vi "Sequencer - Create Sequence.vi"(0 "Error In":errorcluster) -> (8 "Error Out":errorcluster)   [LabVIEW 2011]
uses:
  <vilib>/Utility/file.llb/Read From Spreadsheet File (string).vi
  <vilib>/Utility/file.llb/Write To Spreadsheet File (string).vi
  Controls/Init-Write-Read.ctl
panel:
  in  "Tab":enum32{"EDIT", "RUN"}(tab)
  in  "BG Process":bool
  in  "Ready":bool
  in  "Load":bool
  in  "Save Button":bool
  in  "Stop Button":bool
  in  "Remove Step":bool
  in  "Down Button":bool
  in  "Up Button":bool
  in  "Add Step":bool
  in  "Sequence":i32(listbox)=1
  in  "Steps":i32(listbox)=1
  in  "NewStep":bool
  in  "Confirm Sequence":i32(listbox)=1
  in  "Cancel":bool
  in  "Run":bool
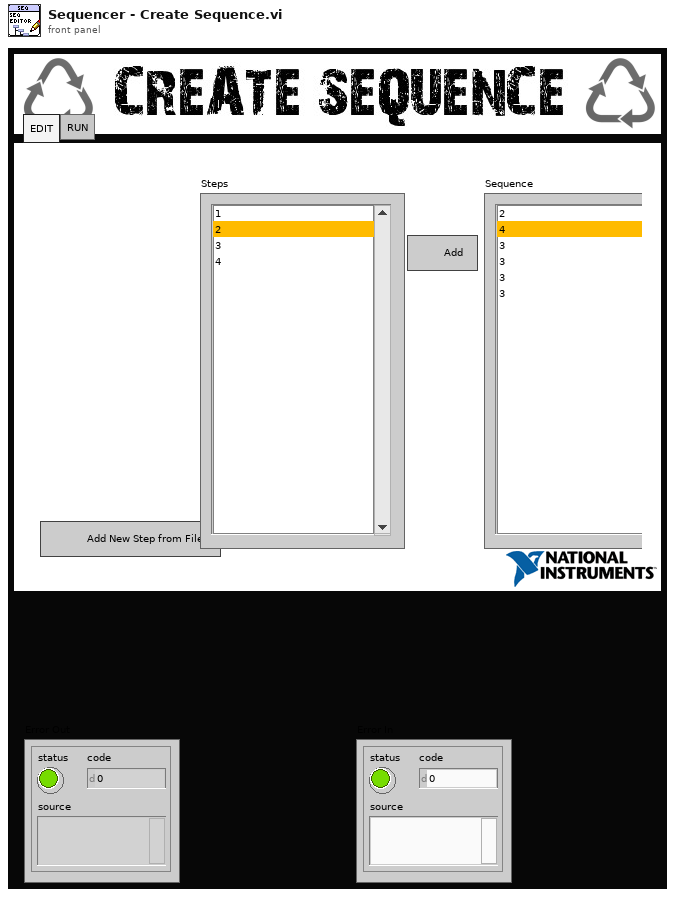
[diagram p1: front panel]
types:
  T1 = typedef "Init-Write-Read.ctl" = enum16{"INIT", "WRITE", "READ", "READ ALL"}
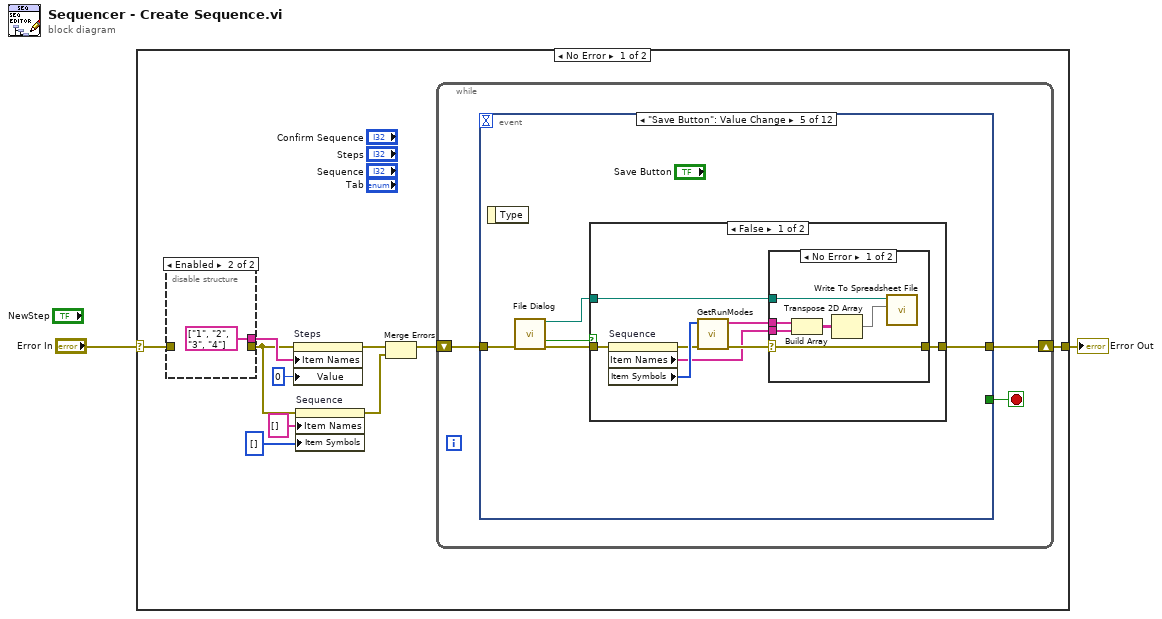
[diagram p0: block diagram]
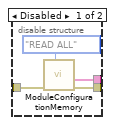
[diagram p2: hidden frame]
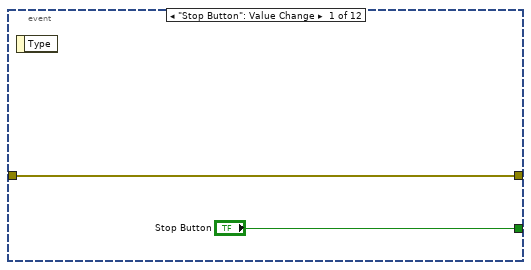
[diagram p3: hidden frame]
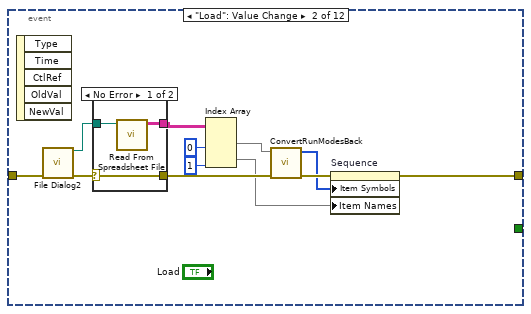
[diagram p4: hidden frame]
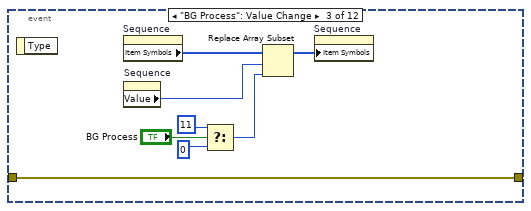
[diagram p6: hidden frame]
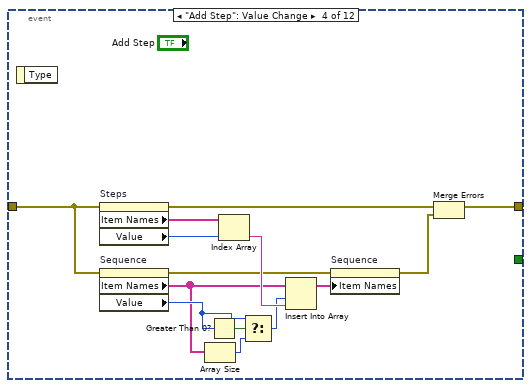
[diagram p7: hidden frame]
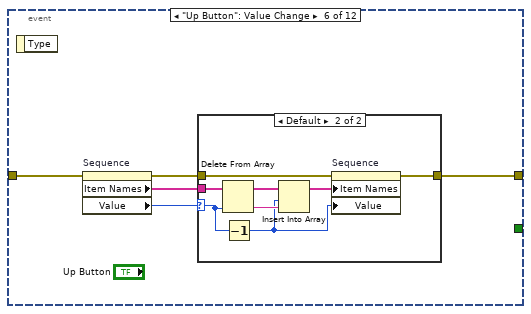
[diagram p10: hidden frame]
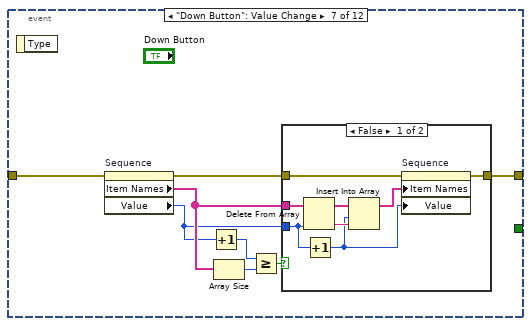
[diagram p12: hidden frame]
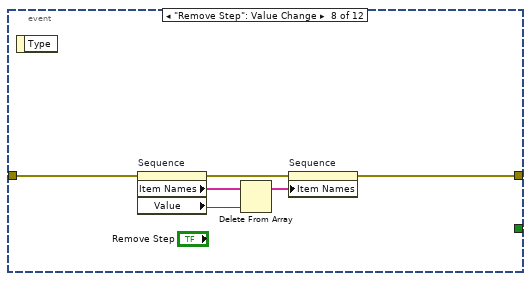
[diagram p14: hidden frame]
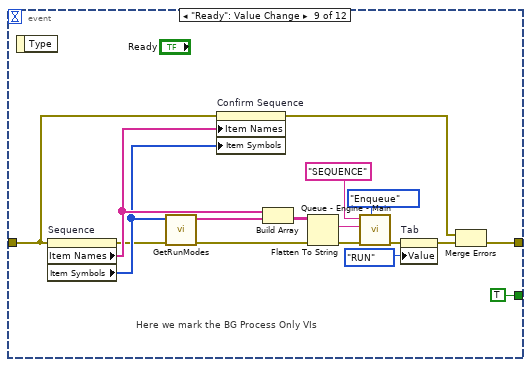
[diagram p15: hidden frame]
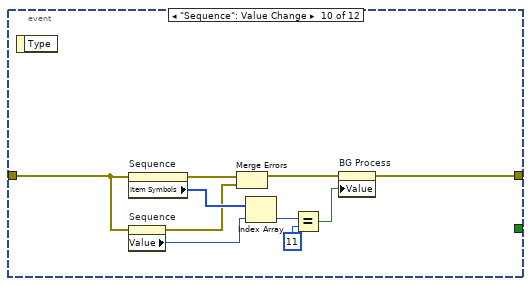
[diagram p16: hidden frame]
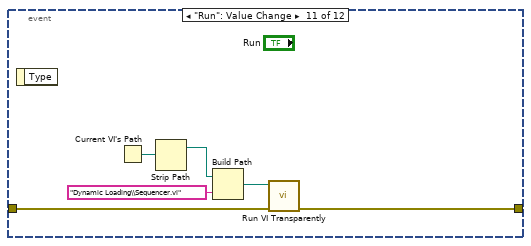
[diagram p17: hidden frame]
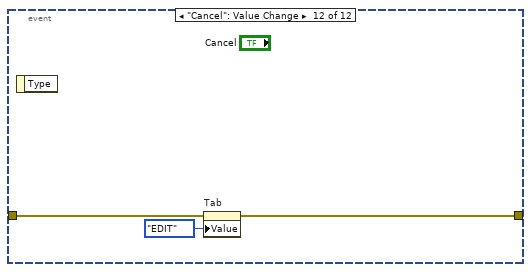
[diagram p18: hidden frame]
diagram:
  n1 = case shown="No Error" "Error In" {
    selector: "Error In" -> [w4 w155]
    tunnel: [w5 w155] -> w2
    frame No Error {
      n2 = disable-structure shown="Enabled" {
        disable-tunnel: [w16 string[] ["1", "2", "3", "4"] ("All Variables Out")] -> w10
        disable-tunnel: [w15 _] -> w9
        disable-tunnel: w4 -> [w14 _]
        frame Disabled {
          n3 = call "ModuleConfigurationMemory.vi"("Operation"=Init-Write-Read."READ ALL", "Error In"=w14) -> ("Error Out"=w15:errorcluster, "All Variables Out"=w16:string[])  [unwired: 5 in, 3 out]
        }
        frame Enabled {
        }
      }
      n4 = property on="Steps" class="LstBox (strict)"(error in=w9, "Item Names"=w10, "Value"=0 ("Steps")) -> (error out=w8:errorcluster)  [unwired: 1 in, 1 out]
      n5 = property on="Sequence" class="LstBox (strict)"(error in=w9, "Item Names"=string[] [], "Item Symbols"=i32[] []) -> (error out=w6:errorcluster)  [unwired: 1 in, 1 out]
      n6 = Merge Errors(w8, w6) -> (w7:errorcluster)
      n7 = while {
        shift-right: [w18] -> w5
        shift-left: w7 -> [w19]
        stop <- w20 stop-if-true
        n8 = event shown="[4] \"Save Button\": Value Change" {
          selector: _ -> [_ _ _ _ _ _ _ _ _ _ _ _]
          dyn-events: _ -> [_ _ _ _ _ _ _ _ _ _ _ _]
          timeout: _ -> [_ _ _ _ _ _ _ _ _ _ _ _]
          tunnel: ["Stop Button" _ _ _ _ _ _ _ TRUE ("Stop Button") _ _ _] -> w20
          tunnel: w19 -> [w21 w31 w43 w51 w62 w83 w97 w114 w126 w140 w151 w153]
          tunnel: [w21 w34 w43 w47 w61 w82 w96 w113 w124 w139 w150 w152] -> w18
          event "Stop Button": Value Change {
            n9 = event-data() -> ()  [unwired: 1 in, 1 out]
          }
          event "Load": Value Change {
            n10 = event-data() -> ()  [unwired: 1 in, 5 out]
            n11 = call "File Dialog2"("error in"=w31) -> ("selected path"=w28:path, "error out"=w30:errorcluster)  [unwired: 11 in, 2 out]
            n12 = case shown="No Error" w30 {
              selector: w30 -> [w37 w38]
              tunnel: [w37 w38] -> w29
              tunnel: w28 -> [w36 _]
              tunnel: [w35 _] -> w27
              frame No Error {
                n13 = call-poly <vilib>:"Read From Spreadsheet File.vi"("file path (dialog if empty)"=w36) -> ("all rows"=w35:string[][])  [unwired: 6 in, 4 out]
              }
              frame Error {
              }
            }
            n14 = Index Array(array=w27, index (col) #1=0 ("disabled index (col)"), index (col) #2=1 ("disabled index (col)")) -> (element #1=w24:string[], element #2=w23:string[])  [unwired: 2 in]
            n15 = call "ConvertRunModesBack.vi"("Error In"=w29, "Run Modes in"=w24) -> ("Error Out"=w33:errorcluster, "Item Symbols Out"=w32:i32[])  [unwired: 8 in]
            n16 = property on="Sequence" class="LstBox (strict)"(error in=w33, "Item Symbols"=w32, "Item Names"=w23) -> (error out=w34:errorcluster)  [unwired: 1 in, 1 out]
          }
          event "BG Process": Value Change {
            n17 = event-data() -> ()  [unwired: 1 in, 1 out]
            n18 = property on="Sequence" class="LstBox (strict)"() -> ("Item Symbols"=w46:i32[])  [unwired: 2 in, 2 out]
            n19 = property on="Sequence" class="LstBox (strict)"() -> ("Value"=w45:i32)  [unwired: 2 in, 2 out]
            n20 = Select(t=11 ("y"), s="BG Process", f=0) -> (s? t:f=w39:i32)
            n21 = Replace Array Subset(array=w46, new element=w39, index=w45) -> (w44:i32[])
            n22 = property on="Sequence" class="LstBox (strict)"("Item Symbols"=w44) -> ()  [unwired: 2 in, 2 out]
          }
          event "Add Step": Value Change {
            n23 = event-data() -> ()  [unwired: 1 in, 1 out]
            n24 = property on="Steps" class="LstBox (strict)"(error in=w51) -> (error out=w49:errorcluster, "Item Names"=w60:string[], "Value"=w59:i32)  [unwired: 1 in, 1 out]
            n25 = property on="Sequence" class="LstBox (strict)"(error in=w51) -> (error out=w50:errorcluster, "Item Names"=w53:string[], "Value"=w55:i32)  [unwired: 1 in, 1 out]
            n26 = Array Size(array=w53) -> (size(s)=w52:i32)
            n27 = Greater Than 0?(x=w55) -> (x > 0?=w56:bool)
            n28 = Index Array(array=w60, index=w59) -> (element=w58:string)
            n29 = Select(t=w55, s=w56, f=w52) -> (s? t:f=w54:i32)
            n30 = Insert Into Array(array=w53, index=w54, new element=w58) -> (w57:string[])
            n31 = property on="Sequence" class="LstBox (strict)"(error in=w50, "Item Names"=w57) -> (error out=w48:errorcluster)  [unwired: 1 in, 1 out]
            n32 = Merge Errors(w49, w48) -> (w47:errorcluster)
          }
          event "Save Button": Value Change {
            n33 = event-data() -> ()  [unwired: 1 in, 1 out]
            n34 = call "File Dialog"("error in"=w62) -> ("selected path"=w63:path, "cancelled"=w65:bool, "error out"=w64:errorcluster)  [unwired: 11 in, 1 out]
            n35 = case shown="False" w65 {
              tunnel: w64 -> [w73 w81]
              tunnel: w63 -> [w68 _]
              tunnel: [w69 w81] -> w61
              frame False {
                n36 = property on="Sequence" class="LstBox (strict)"(error in=w73) -> (error out=w71:errorcluster, "Item Names"=w66:string[], "Item Symbols"=w72:i32[])  [unwired: 1 in, 1 out]
                n37 = call "GetRunModes.vi"("Error In"=w71, "Item Symbols In"=w72) -> ("Error Out"=w70:errorcluster, "Run Modes Out"=w67:string[])  [unwired: 8 in]
                n38 = case shown="No Error" w70 {
                  selector: w70 -> [w79 w80]
                  tunnel: [w79 w80] -> w69
                  tunnel: w68 -> [w78 _]
                  tunnel: w67 -> [w77 _]
                  tunnel: w66 -> [w76 _]
                  frame No Error {
                    n39 = Build Array(w77, w76) -> (w75:string[][])
                    n40 = Transpose 2D Array(2D array=w75) -> (transposed array=w74:string[][])
                    n41 = call-poly <vilib>:"Write To Spreadsheet File.vi"("2D data"=w74, "file path (dialog if empty)"=w78) -> ()  [unwired: 6 in, 1 out]
                  }
                  frame Error {
                  }
                }
              }
              frame True {
              }
            }
          }
          event "Up Button": Value Change {
            n42 = event-data() -> ()  [unwired: 1 in, 1 out]
            n43 = property on="Sequence" class="LstBox (strict)"(error in=w83) -> (error out=w85:errorcluster, "Item Names"=w86:string[], "Value"=w84:i32)  [unwired: 1 in, 1 out]
            n44 = case shown="Default" w84 {
              selector: w84 -> [_ w89]
              tunnel: w86 -> [_ w95]
              tunnel: w85 -> [w87 w91]
              tunnel: [w87 w88] -> w82
              frame 0 {
              }
              frame Default {
                n45 = Delete From Array(array=w95, index=w89) -> (deleted portion=w93:string, array with subset deleted=w94:string[])  [unwired: 1 in]
                n46 = Decrement(x=w89) -> (x-1=w90:i32)
                n47 = Insert Into Array(array=w94, index=w90, new element=w93) -> (w92:string[])
                n48 = property on="Sequence" class="LstBox (strict)"(error in=w91, "Item Names"=w92, "Value"=w90) -> (error out=w88:errorcluster)  [unwired: 1 in, 1 out]
              }
            }
          }
          event "Down Button": Value Change {
            n49 = event-data() -> ()  [unwired: 1 in, 1 out]
            n50 = property on="Sequence" class="LstBox (strict)"(error in=w97) -> (error out=w103:errorcluster, "Item Names"=w102:string[], "Value"=w100:i32)  [unwired: 1 in, 1 out]
            n51 = Increment(x=w100) -> (x+1=w98:i32)
            n52 = Array Size(array=w102) -> (size(s)=w101:i32)
            n53 = Greater Or Equal?(x=w98, y=w101) -> (x >= y?=w99:bool)
            n54 = case shown="False" w99 {
              tunnel: w103 -> [w109 w112]
              tunnel: w102 -> [w108 _]
              tunnel: w100 -> [w106 _]
              tunnel: [w104 w112] -> w96
              frame False {
                n55 = Delete From Array(array=w108, index=w106) -> (deleted portion=w110:string, array with subset deleted=w111:string[])  [unwired: 1 in]
                n56 = Increment(x=w106) -> (x+1=w107:i32)
                n57 = Insert Into Array(array=w111, index=w107, new element=w110) -> (w105:string[])
                n58 = property on="Sequence" class="LstBox (strict)"(error in=w109, "Item Names"=w105, "Value"=w107) -> (error out=w104:errorcluster)  [unwired: 1 in, 1 out]
              }
              frame True {
              }
            }
          }
          event "Remove Step": Value Change {
            n59 = event-data() -> ()  [unwired: 1 in, 1 out]
            n60 = property on="Sequence" class="LstBox (strict)"(error in=w114) -> (error out=w116:errorcluster, "Item Names"=w118:string[], "Value"=w115:i32)  [unwired: 1 in, 1 out]
            n61 = Delete From Array(array=w118, index=w115) -> (array with subset deleted=w117:string[])  [unwired: 1 in, 1 out]
            n62 = property on="Sequence" class="LstBox (strict)"(error in=w116, "Item Names"=w117) -> (error out=w113:errorcluster)  [unwired: 1 in, 1 out]
          }
          event "Ready": Value Change {
            # "Here we mark the BG Process Only VIs"
            n63 = event-data() -> ()  [unwired: 1 in, 1 out]
            n64 = property on="Sequence" class="LstBox (strict)"(error in=w126) -> (error out=w120:errorcluster, "Item Names"=w127:string[], "Item Symbols"=w122:i32[])  [unwired: 1 in, 1 out]
            n65 = call "GetRunModes.vi"("Error In"=w120, "Item Symbols In"=w122) -> ("Error Out"=w119:errorcluster, "Run Modes Out"=w121:string[])  [unwired: 8 in]
            n66 = property on="Confirm Sequence" class="LstBox (strict)"(error in=w126, "Item Names"=w127, "Item Symbols"=w122) -> (error out=w123:errorcluster)  [unwired: 1 in, 1 out]
            n67 = Build Array(w127, w121) -> (w130:string[][])
            n68 = Flatten To String(anything=w130, error in (no error)=w119) -> (data string=w132:string, error out=w131:errorcluster)  [unwired: 2 in, 1 out]
            n69 = call "Queue - Engine - Main.vi"("Operation"=enum16{"Enqueue", "Dequeue", "Flush", "Release"}."Enqueue", "error in"=w131, "Queue Data In"=w132, "Queue Name In"="SEQUENCE") -> ("error out"=w129:errorcluster)  [unwired: 5 in, 2 out]
            n70 = property on="Tab" class="TabCtl (strict)"(error in=w129, "Value"=enum32{"EDIT", "RUN"}."RUN" ("Tab Control")) -> (error out=w125:errorcluster)  [unwired: 1 in, 1 out]
            n71 = Merge Errors(w123, w125) -> (w124:errorcluster)
          }
          event "Sequence": Value Change {
            n72 = event-data() -> ()  [unwired: 1 in, 1 out]
            n73 = property on="Sequence" class="LstBox (strict)"(error in=w140) -> (error out=w138:errorcluster, "Item Symbols"=w145:i32[])  [unwired: 1 in, 1 out]
            n74 = property on="Sequence" class="LstBox (strict)"(error in=w140) -> (error out=w137:errorcluster, "Value"=w144:i32)  [unwired: 1 in, 1 out]
            n75 = Merge Errors(w138, w137) -> (w136:errorcluster)
            n76 = Index Array(array=w145, index=w144) -> (element=w143:i32)
            n77 = Equal?(x=w143, y=11) -> (x = y?=w141:bool)
            n78 = property on="BG Process" class="Bool (strict)"(error in=w136, "Value"=w141) -> (error out=w139:errorcluster)  [unwired: 1 in, 1 out]
          }
          event "Run": Value Change {
            n79 = event-data() -> ()  [unwired: 1 in, 1 out]
            n80 = Current VI's Path() -> (path=w149:path)
            n81 = Strip Path(path=w149) -> (stripped path=w148:path)  [unwired: 1 out]
            n82 = Build Path(base path=w148, name or relative path="Dynamic Loading\\Sequencer.vi") -> (appended path=w146:path)
            n83 = call "Run VI Transparently.vi"("error in"=w151, "vi path"=w146) -> ("error out"=w150:errorcluster)  [unwired: 9 in]
          }
          event "Cancel": Value Change {
            n84 = event-data() -> ()  [unwired: 1 in, 1 out]
            n85 = property on="Tab" class="TabCtl (strict)"(error in=w153, "Value"=enum32{"EDIT", "RUN"}."EDIT" ("Tab Control")) -> (error out=w152:errorcluster)  [unwired: 1 in, 1 out]
          }
        }
      }
    }
    frame Error {
    }
  }
  "Error Out" <- w2
